vi "cwlaserSetPower.vi"(1 "power (mW)":dbl, 2 "wavelength":dbl) -> (0 "success":bool)   [LabVIEW 2017]
uses:
  globalDevices.vi
panel:
  out "set string":string
  out "read buffer":string
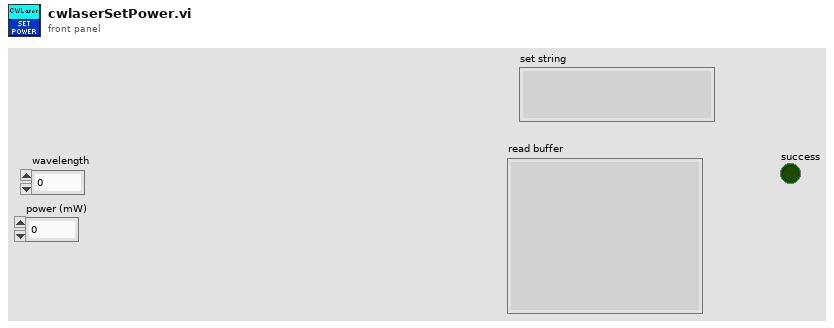
[diagram p1: front panel]
types:
  T1 = cluster{"serialPort":refnum<visa-resource-name>, "error":errorcluster, "power (mW)":dbl, "wavelength (nm)":dbl, "type":string}[]
  T2 = cluster{"serialPort":refnum<visa-resource-name>, "error":errorcluster, "power (mW)":dbl, "wavelength (nm)":dbl, "type":string}
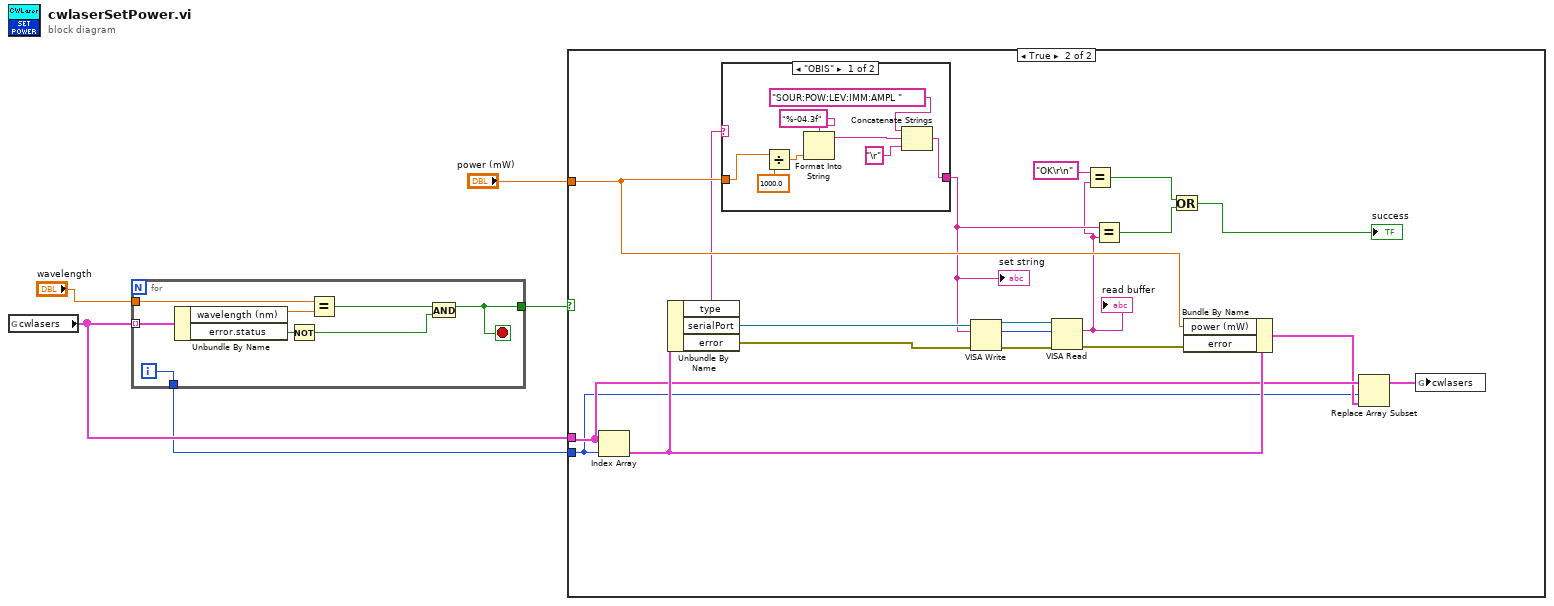
[diagram p0: block diagram]
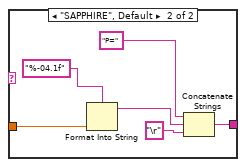
[diagram p3: hidden frame]
diagram:
  n1 = global read "globalDevices.vi" "cwlasers"() -> (w2:T1)
  n2 = for {
    tunnel: w2 -> [w13] mode=indexing
    tunnel: "wavelength" -> [w11]
    tunnel: [w9] -> w3
    tunnel: [w6] -> w1
    i -> [w6]
    stop <- w9 stop-if-true
    n3 = Unbundle By Name(w13) -> ("wavelength (nm)"=w12:dbl, "error.status"=w7:bool)
    n4 = Not(x=w7) -> (.not. x?=w8:bool)
    n5 = Equal?(x=w11, y=w12) -> (x = y?=w10:bool)
    n6 = And(x=w10, y=w8) -> (x .and. y?=w9:bool)
  }
  n7 = case shown="True" w3 {
    tunnel: "power (mW)" -> [_ w22]
    tunnel: w2 -> [_ w26]
    tunnel: w1 -> [_ w24]
    frame False {
    }
    frame True {
      n8 = Index Array(array=w26, index=w24) -> (element=w28:T2)
      n9 = Unbundle By Name(w28) -> ("type"=w20:string, "serialPort"=w32:refnum<visa-resource-name>, "error"=w31:errorcluster)
      n10 = case shown="\"OBIS\"" w20 {
        tunnel: w22 -> [w33 w42]
        tunnel: [w34 w41] -> w18
        frame "OBIS" {
          n11 = Divide(x=w33, y=1000.0) -> (x/y=w39:dbl)
          n12 = Format Into String(format string="%-04.3f", w39) -> (resulting string=w40:string)  [unwired: 2 in, 1 out]
          n13 = Concatenate Strings("SOUR:POW:LEV:IMM:AMPL " ("string"), w40, "\r" ("string")) -> (w34:string)
        }
        frame "SAPPHIRE", Default {
          n14 = Format Into String(format string="%-04.1f", w42) -> (resulting string=w44:string)  [unwired: 2 in, 1 out]
          n15 = Concatenate Strings("P=" ("OutString"), w44, "\r") -> (w41:string)
        }
      }
      "set string" <- w18
      n16 = VISA Write(VISA resource name=w32, write buffer=w18, error in (no error)=w31) -> (VISA resource name out=w30:refnum<visa-resource-name>, return count=w21:u32, error out=w29:errorcluster)
      n17 = VISA Read(VISA resource name=w30, byte count=w21, error in (no error)=w29) -> (read buffer=w14:string, error out=w27:errorcluster)  [unwired: 2 out]
      "read buffer" <- w14
      n18 = Equal?(x="OK\r\n", y=w14) -> (x = y?=w15:bool)
      n19 = Equal?(x=w18, y=w14) -> (x = y?=w17:bool)
      n20 = Or(x=w15, y=w17) -> (x .or. y?=→"success":bool)
      n21 = Bundle By Name(cluster=w28, "power (mW)"=w22, "error"=w27) -> (w25:T2)
      n22 = Replace Array Subset(array=w26, new element=w25, index=w24) -> (w23:T1)
      n23 = global write "globalDevices.vi" "cwlasers"(w23) -> ()
    }
  }
